vi "Stop Error Loop.vi"(8 "Error In":errorcluster) -> (0 "Error Out":errorcluster)   [LabVIEW 2019, in "TSC Error.lvlib"]
doc: "This VI will send the stop message to the error loop.\n\n<b>Note:</b> this should be called as a way to finish the error loop in the application and should be called when it is time to shut down\n\n<b>Code Developed By:</b>\nDaniel Coons\nTechnology Service Corporation\n1983 S Liberty Drive\nBloomington, IN 47403\nwww.tsc.com\\atcs"
uses:
  TSC Error.lvlib
  _Messages/ERROR_Stop/ERROR_Stop.lvclass
  C:/Development/Open Source/tsc-error-library/_Messages/Error/Error.lvclass
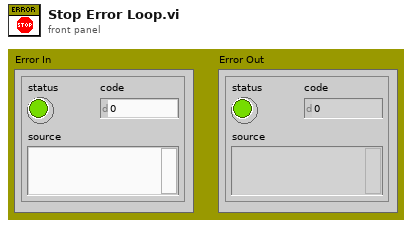
[diagram p1: front panel]
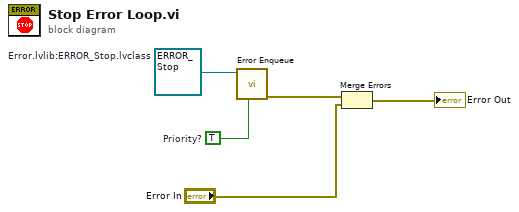
[diagram p0: block diagram]
diagram:
  w3 = TRUE  # Priority?
  w5 = refnum<class "ERROR_Stop.lvclass"> refnum  # Error.lvlib:ERROR_Stop.lvclass
  n1 = call "Error Enqueue.vi"("Priority?"=w3, "Error Message in"=w5) -> ("error out"=w4:errorcluster)  [unwired: 8 in, 1 out]
  n2 = Merge Errors(w4, "Error In") -> (→"Error Out":errorcluster)
